vi "Separate_Prices.vi"(11 "Frame":string) -> (3 "Base Price":T1={"DELICATE"=0.0, "LOW"=0.0, "MEDIUM"=0.5, "HIGH"=0.25} {"HIGH" min=0.0 max=9.75 step=0.25; "MEDIUM" min=0.0 max=9.75 step=0.25; "LOW" min=0.0 max=9.75 step=0.25; "DELICATE" min=0.0 max=9.75 step=0.25})   [LabVIEW 2023]
panel:
  out "error out":errorcluster
  in  "error in":errorcluster
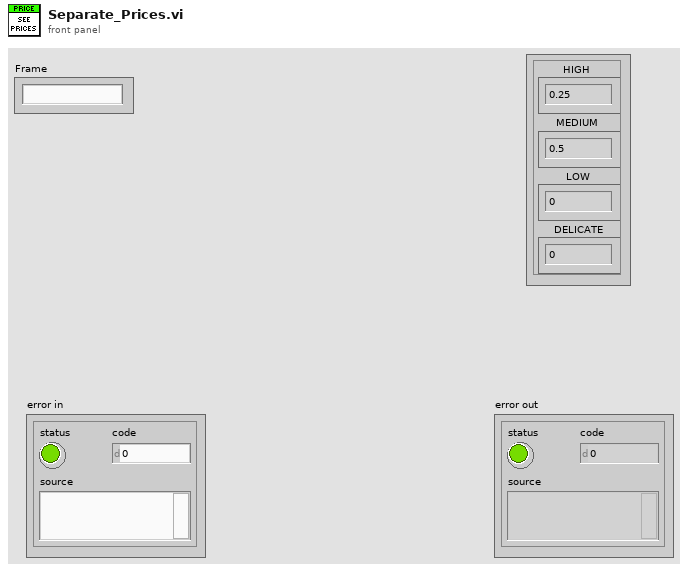
[diagram p1: front panel]
types:
  T1 = cluster{"DELICATE":dbl, "LOW":dbl, "MEDIUM":dbl, "HIGH":dbl}
  T2 = cluster{"Delicates":dbl, "Low":dbl, "Medium":dbl, "High":dbl}
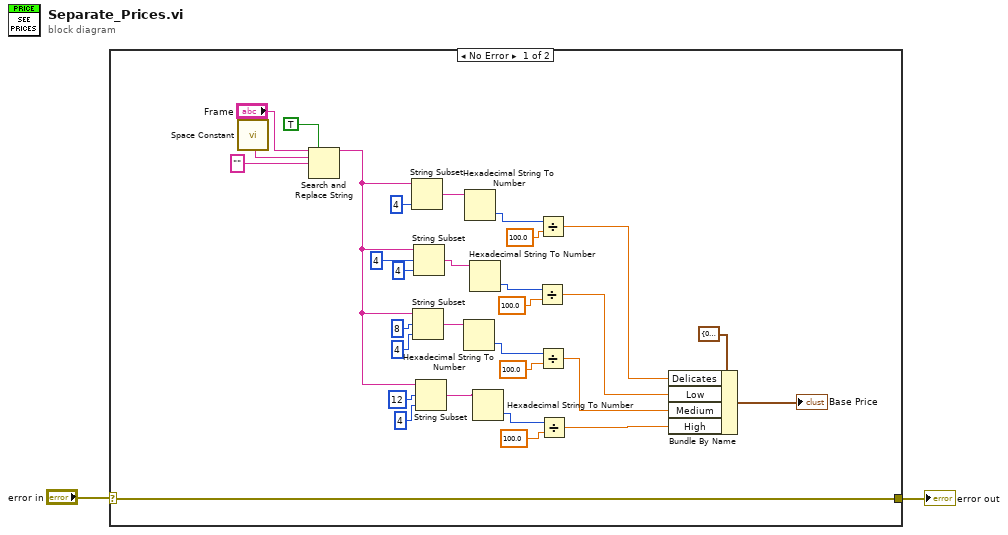
[diagram p0: block diagram]
diagram:
  n1 = case shown="No Error" "error in" {
    selector: "error in" -> [w11 w34]
    tunnel: [w11 w34] -> w1
    frame No Error {
      n2 = call <vilib>:"Space Constant.vi"() -> ("String"=w30:string)
      n3 = Search and Replace String(replace all?=TRUE ("replace all? (F)"), input string="Frame", search string=w30, replace string="" ("replace string (\"\")")) -> (result string=w22:string)  [unwired: 4 in, 3 out]
      n4 = String Subset(string=w22, length (rest)=4 ("length (rest)")) -> (substring=w10:string)  [unwired: 1 in]
      n5 = String Subset(string=w22, offset (0)=8, length (rest)=4 ("length (rest)")) -> (substring=w6:string)
      n6 = String Subset(string=w22, offset (0)=4, length (rest)=4 ("length (rest)")) -> (substring=w8:string)
      n7 = String Subset(string=w22, offset (0)=12, length (rest)=4 ("length (rest)")) -> (substring=w4:string)
      n8 = Hexadecimal String To Number(string=w6) -> (number=w5:u32)  [unwired: 2 in, 1 out]
      n9 = Hexadecimal String To Number(string=w10) -> (number=w9:u32)  [unwired: 2 in, 1 out]
      n10 = Hexadecimal String To Number(string=w8) -> (number=w7:u32)  [unwired: 2 in, 1 out]
      n11 = Hexadecimal String To Number(string=w4) -> (number=w3:u32)  [unwired: 2 in, 1 out]
      n12 = Divide(x=w7, y=100.0) -> (x/y=w15:dbl)
      n13 = Divide(x=w9, y=100.0) -> (x/y=w16:dbl)
      n14 = Divide(x=w5, y=100.0) -> (x/y=w14:dbl)
      n15 = Divide(x=w3, y=100.0) -> (x/y=w13:dbl)
      n16 = Bundle By Name(cluster=T2 {"Delicates"=0.0, "Low"=0.0, "Medium"=0.0, "High"=0.0}, "Delicates"=w16, "Low"=w15, "Medium"=w14, "High"=w13) -> (→"Base Price":T2)
    }
    frame Error {
    }
  }
  "error out" <- w1
